vi "LedOff.vi"(8 "error in (no error)":errorcluster) -> (0 "error out":errorcluster)   [LabVIEW 2015, in "ESLSCDLL.lvlib"]
uses:
  ESLSCDLL.lvlib
  Globals.vi
  ESLSCDLL.dll
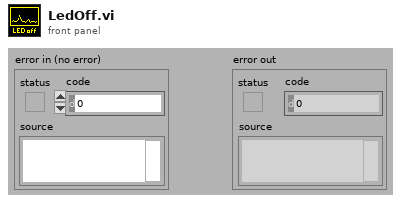
[diagram p1: front panel]
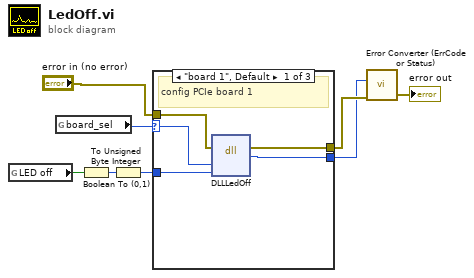
[diagram p0: block diagram]
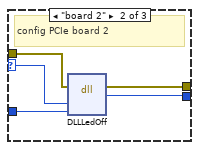
[diagram p2: hidden frame]
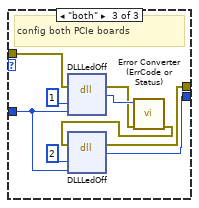
[diagram p3: hidden frame]
diagram:
  n1 = global read "Globals.vi" "LED off"() -> (w1:bool)
  n2 = global read "Globals.vi" "board_sel"() -> (w2:enum32{"0", "board 1", "board 2", "both"})
  n3 = Boolean To (0,1)(Boolean=w1) -> (0, 1=w7:i16)
  n4 = To Unsigned Byte Integer(number=w7) -> (unsigned 8bit integer=w8:u8)
  n5 = case shown="\"board 1\", Default" w2 {
    selector: w2 -> [w13 w17 _]
    tunnel: w8 -> [w12 w18 w25]
    tunnel: "error in (no error)" -> [w11 w14 w24]
    tunnel: [w10 w15 w20] -> w4
    tunnel: [w9 w16 w19] -> w3
    frame "board 1", Default {
      # "config PCIe board 1"
      n6 = dll-call lib="C:/ENTW/PCIE/LV64/board.vis/ESLSCDLL.dll" fn="DLLLedOff" ("lwlscdll.dll:DLLSetADAmpRed")(error in=w11, "drv"=w13, "LED_OFF"=w12) -> (error out=w10:errorcluster, "es_status_codes"=w9:i32)  [unwired: 4 in, 1 out]
    }
    frame "board 2" {
      # "config PCIe board 2"
      n7 = dll-call lib="C:/ENTW/PCIE/LV64/board.vis/ESLSCDLL.dll" fn="DLLLedOff" ("lwlscdll.dll:DLLSetADAmpRed")(error in=w14, "drv"=w17, "LED_OFF"=w18) -> (error out=w15:errorcluster, "es_status_codes"=w16:i32)  [unwired: 4 in, 1 out]
    }
    frame "both" {
      # "config both PCIe boards"
      n8 = dll-call lib="C:/ENTW/PCIE/LV64/board.vis/ESLSCDLL.dll" fn="DLLLedOff" ("lwlscdll.dll:DLLSetADAmpRed")(error in=w24, "drv"=u32 1, "LED_OFF"=w25) -> (error out=w22:errorcluster, "es_status_codes"=w23:i32)  [unwired: 4 in, 1 out]
      n9 = call "Error Converter (ErrCode or Status).vi"("error in (no error)"=w22, "error code"=w23) -> ("error out"=w21:errorcluster)  [unwired: 9 in]
      n10 = dll-call lib="C:/ENTW/PCIE/LV64/board.vis/ESLSCDLL.dll" fn="DLLLedOff" ("lwlscdll.dll:DLLSetADAmpRed")(error in=w21, "drv"=u32 2, "LED_OFF"=w25) -> (error out=w20:errorcluster, "es_status_codes"=w19:i32)  [unwired: 4 in, 1 out]
    }
  }
  n11 = call "Error Converter (ErrCode or Status).vi"("error in (no error)"=w4, "error code"=w3) -> ("error out"=→"error out":errorcluster)  [unwired: 9 in]
